vi "rojovivo.vi"() -> ()   [LabVIEW 2020]
uses:
  Downloads/Vending Machine/Case Selector.ctl
panel:
  in  "Estado":string
  out "Total":dbl
  out "Change":dbl
  out "Product Delivered":bool
  in  "MONEDA":cluster{"$ 10":bool, "$ 20":bool}
  in  "PRODUCTOS":T1
  in  "Stop":bool
  # "Price Per Item"
  # "Add Money Here"
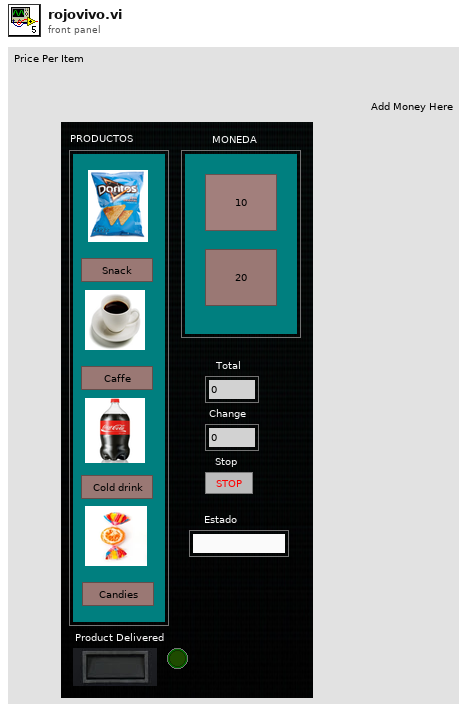
[diagram p1: front panel]
types:
  T1 = cluster{"Sanack":bool, "Caffe":bool, "Cold drink":bool, "Candies":bool}
  T2 = typedef "Case Selector.ctl" = enum16{"Return Change", "Select Product", "Add Money", "Waiting", "Start-Up", "Dispense Product"}
  T3 = enum16{"Return Change", "Select Product", "Add Money", "Waiting", "Start-Up"}
  T4 = cluster{"Cherry Rush":bool, "Lime Fizz":bool, "Orange Blast":bool, "Mr. Fizzle":bool}
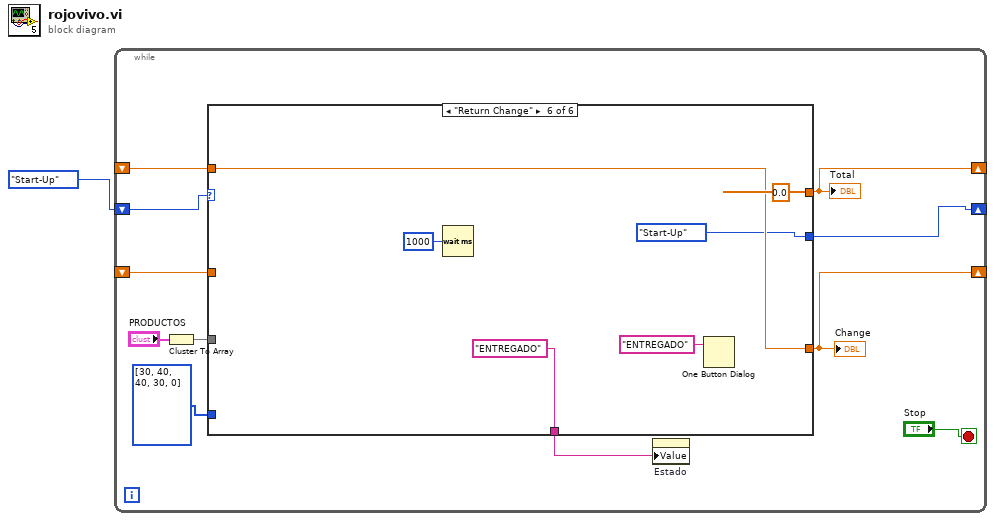
[diagram p0: block diagram]
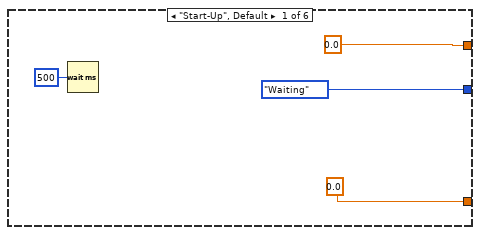
[diagram p2: hidden frame]
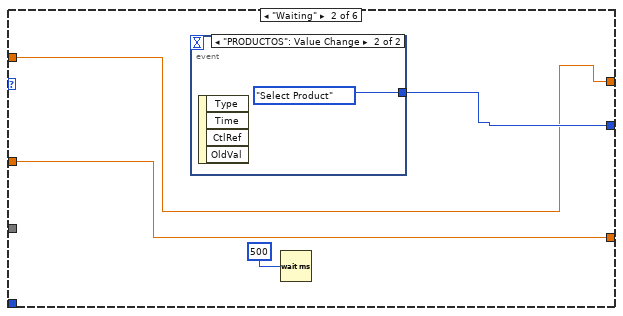
[diagram p3: hidden frame]
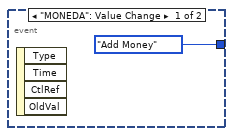
[diagram p4: hidden frame]
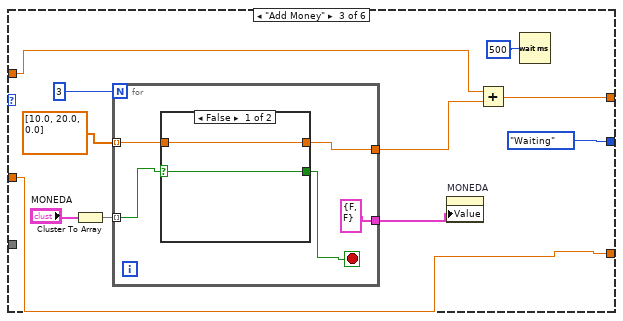
[diagram p5: hidden frame]
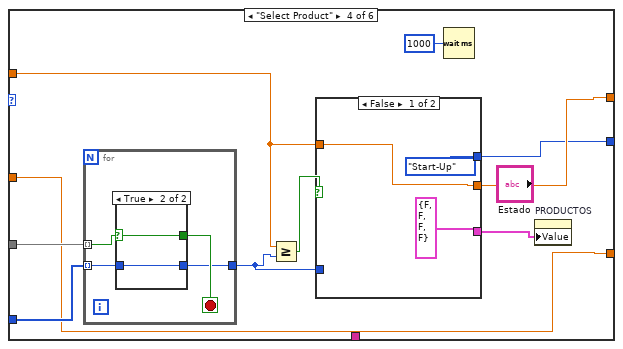
[diagram p7: hidden frame]
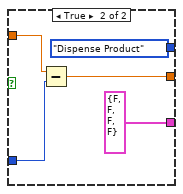
[diagram p8: hidden frame]
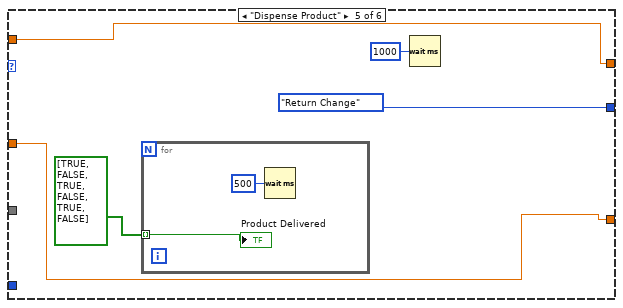
[diagram p10: hidden frame]
diagram:
  n1 = while {
    shift-right: [w11] -> _
    shift-left: Case_Selector."Start-Up" ("Enum") -> [w12]
    shift-right: [w6] -> _
    shift-left: _ -> [w7]
    shift-right: [w5] -> _
    shift-left: _ -> [w4]
    stop <- "Stop" stop-if-true
    n2 = Cluster To Array(cluster="PRODUCTOS") -> (array=w9:bool[])
    n3 = case shown="\"Return Change\"" w12 {
      tunnel: [T3."Waiting" ("Enum") w20 Case_Selector."Waiting" ("Enum") w46 Case_Selector."Return Change" ("Enum") Case_Selector."Start-Up" ("Enum")] -> w11
      tunnel: [0.0 w18 w27 w47 w73 0.0] -> w6
      tunnel: w9 -> [_ _ _ w52 _ _]
      tunnel: i32[] [30, 40, 40, 30, 0] -> [_ _ _ w51 _ _]
      tunnel: w7 -> [_ w18 w25 w48 w73 w80]
      tunnel: [0.0 w19 w28 w45 w71 w80] -> w5
      tunnel: w4 -> [_ w19 w28 w45 w71 _]
      tunnel: [_ _ _ _ _ "ENTREGADO" ("Estado")] -> w2
      frame "Start-Up", Default {
        n4 = Wait (ms)(milliseconds to wait=u32 500) -> ()  [unwired: 1 out]
      }
      frame "Waiting" {
        n5 = event shown="[1] \"PRODUCTOS\": Value Change" {
          selector: _ -> [_ _]
          dyn-events: _ -> [_ _]
          timeout: _ -> [_ _]
          tunnel: [Case_Selector."Add Money" ("Enum") T3."Select Product" ("Enum")] -> w20
          event "MONEDA": Value Change {
            n6 = event-data() -> ()  [unwired: 1 in, 4 out]
          }
          event "PRODUCTOS": Value Change {
            n7 = event-data() -> ()  [unwired: 1 in, 4 out]
          }
        }
        n8 = Wait (ms)(milliseconds to wait=u32 500) -> ()  [unwired: 1 out]
      }
      frame "Add Money" {
        n9 = Cluster To Array(cluster="MONEDA") -> (array=w31:bool[])
        n10 = for {
          N: 3 -> [_]
          tunnel: w31 -> [w38] mode=indexing
          tunnel: dbl[] [10.0, 20.0, 0.0] -> [w37] mode=indexing
          tunnel: [w36] -> w26
          tunnel: [cluster{"10 Cents":bool, "5 Cents":bool} {"10 Cents"=FALSE, "5 Cents"=FALSE} ("Insert Coins")] -> w24
          stop <- w34 stop-if-true
          n11 = case shown="False" w38 {
            selector: w38 -> [w39 w41]
            tunnel: w37 -> [w40 w42]
            tunnel: [w40 w42] -> w36
            tunnel: [w39 w41] -> w34
            frame False {
            }
            frame True {
            }
          }
        }
        n12 = property on="MONEDA" class="Clust (strict)"("Value"=w24) -> ()  [unwired: 2 in, 2 out]
        n13 = Add(x=w25, y=w26) -> (x+y=w27:dbl)
        n14 = Wait (ms)(milliseconds to wait=u32 500) -> ()  [unwired: 1 out]
      }
      frame "Select Product" {
        n15 = for {
          tunnel: w52 -> [w64] mode=indexing
          tunnel: w51 -> [w62] mode=indexing
          tunnel: [w61] -> w49
          stop <- w63 stop-if-true
          n16 = case shown="True" w64 {
            selector: w64 -> [w66 w68]
            tunnel: [w66 w68] -> w63
            tunnel: w62 -> [w65 w67]
            tunnel: [w65 w67] -> w61
            frame False {
            }
            frame True {
            }
          }
        }
        n17 = Greater Or Equal?(x=w48, y=w49) -> (x >= y?=w50:bool)
        n18 = case shown="False" w50 {
          tunnel: w49 -> [_ w59]
          tunnel: w48 -> [w55 w60]
          tunnel: [w55 w58] -> w47
          tunnel: [Case_Selector."Start-Up" ("Enum") Case_Selector."Dispense Product" ("Enum")] -> w46
          tunnel: [T4 {"Cherry Rush"=FALSE, "Lime Fizz"=FALSE, "Orange Blast"=FALSE, "Mr. Fizzle"=FALSE} ("Choose from \nthese:") T4 {"Cherry Rush"=FALSE, "Lime Fizz"=FALSE, "Orange Blast"=FALSE, "Mr. Fizzle"=FALSE} ("Choose from \nthese:")] -> w43
          frame False {
          }
          frame True {
            n19 = Subtract(x=w60, y=w59) -> (x-y=w58:dbl)
          }
        }
        n20 = Wait (ms)(milliseconds to wait=u32 1000) -> ()  [unwired: 1 out]
        n21 = property on="PRODUCTOS" class="Clust (strict)"("Value"=w43) -> ()  [unwired: 2 in, 2 out]
      }
      frame "Dispense Product" {
        n22 = for {
          tunnel: bool[] [TRUE, FALSE, TRUE, FALSE, TRUE, FALSE] -> [w74] mode=indexing
          n23 = Wait (ms)(milliseconds to wait=u32 500) -> ()  [unwired: 1 out]
          "Product Delivered" <- w74
        }
        n24 = Wait (ms)(milliseconds to wait=u32 1000) -> ()  [unwired: 1 out]
      }
      frame "Return Change" {
        n25 = Wait (ms)(milliseconds to wait=u32 1000) -> ()  [unwired: 1 out]
        n26 = One Button Dialog(message="ENTREGADO") -> ()  [unwired: 1 in, 1 out]
      }
    }
    "Total" <- w6
    "Change" <- w5
    n27 = property on="Estado" class="Str"("Value"=w2) -> ()  [unwired: 2 in, 2 out]
  }
